vi "CalculateErrorOutLeftPosition__slk_mt.vi"(3 "add error configure":T2, 7 "position in":T1, 8 "error in (no error)":errorcluster, 11 "\"error in\" width":u32) -> (0 "error out":errorcluster, 5 "position out":T1)   [LabVIEW 2010, in "Lazyboots Menu Tool.lvlib"]
doc: "Gets error out left position."
uses:
  Library/Lazyboots Menu Tool.lvlib
  TypeDef/TypeDef_AddErrorConfigure__slk_mt.ctl
  <vilib>/Utility/miscctls.llb/LVPositionTypeDef.ctl
panel:
  # "CalculateErrorOutLeftPosition__slk_mt.vi\nGets error out left position.\n\nNOTICE -- YOU MUST LEAVE THIS NOTICE IN PLACE.\n\nCopyright (c) 2011, LIANG LIU Shawn.Liu.cn@gmail.com\nAll rights reserved.\n\nRedistribution and use in source and binary forms, with or without modification, are permitted provided that the following conditions are met:\n-Redistributions of source code must retain the above copyright notice, this list of conditions and the following disclaimer.\n-Redistributions in binary form must reproduce the above copyright notice, this list of conditions and the following disclaimer in the documentation and/or other materials provided with the distribution.\n-Neither the name of the eLp nor the names of its contributors may be used to endorse or promote products derived from this software without specific prior written permission.\n\nTHIS SOFTWARE IS PROVIDED BY THE COPYRIGHT HOLDERS AND CONTRIBUTORS \"AS IS\" AND ANY EXPRESS OR IMPLIED WARRANTIES, INCLUDING, BUT NOT LIMITED TO, THE IMPLIED WARRANTIES OF MERCHANTABILITY AND FITNESS FOR A PARTICULAR PURPOSE ARE DISCLAIMED. IN NO EVENT SHALL THE COPYRIGHT HOLDER OR CONTRIBUTORS BE LIABLE FOR ANY DIRECT, INDIRECT, INCIDENTAL, SPECIAL, EXEMPLARY, OR CONSEQUENTIAL DAMAGES (INCLUDING, BUT NOT LIMITED TO, PROCUREMENT OF SUBSTITUTE GOODS OR SERVICES; LOSS OF USE, DATA, OR PROFITS; OR BUSINESS INTERRUPTION) HOWEVER CAUSED AND ON ANY THEORY OF LIABILITY, WHETHER IN CONTRACT, STRICT LIABILITY, OR TORT (INCLUDING NEGLIGENCE OR OTHERWISE) ARISING IN ANY WAY OUT OF THE USE OF THIS SOFTWARE, EVEN IF ADVISED OF THE POSSIBILITY OF SUCH DAMAGE."
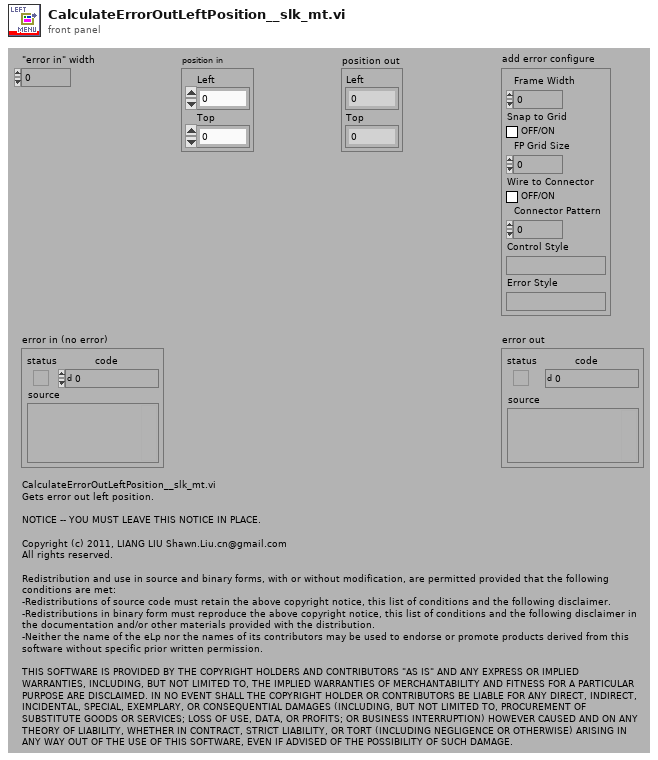
[diagram p1: front panel]
types:
  T1 = typedef "LVPositionTypeDef.ctl" = cluster{"Left":i32, "Top":i32}
  T2 = typedef "Lazyboots Menu Tool.lvlib/TypeDef_AddErrorConfigure__slk_mt.ctl" = cluster{"Frame Width":u32, "Snap to Grid":bool, "FP Grid Size":u32, "Wire to Connector":bool, "Connector Pattern":u32, "Control Style":string, "Error Style":string}
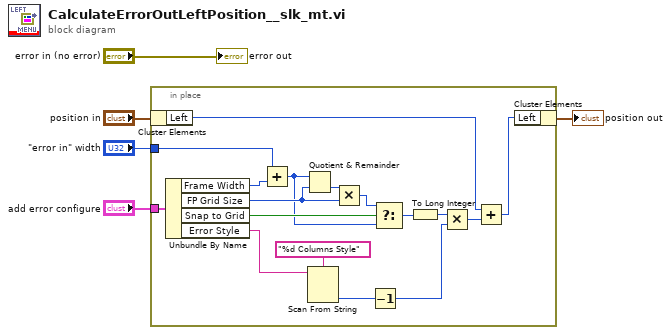
[diagram p0: block diagram]
diagram:
  n1 = in-place {
    in-place-border: "add error configure" -> [w22]
    in-place-border: "\"error in\" width" -> [w13]
    n2 = in-place-cluster #1("position in") -> ("Left"=w16:i32)
    n3 = Unbundle By Name(w22) -> ("Frame Width"=w15:u32, "FP Grid Size"=w14:u32, "Snap to Grid"=w8:bool, "Error Style"=w9:string)
    n4 = Add(x=w13, y=w15) -> (x+y=w7:u32)
    n5 = Quotient & Remainder(x=w7, y=w14) -> (floor(x/y)=w17:u32)  [unwired: 1 out]
    n6 = Scan From String(format string="%d Columns Style", input string=w9) -> (output 1=w19:i32)  [unwired: 3 in, 3 out]
    n7 = Multiply(x=w17, y=w14) -> (x*y=w10:u32)
    n8 = Decrement(x=w19) -> (x-1=w20:i32)
    n9 = Select(t=w10, s=w8, f=w7) -> (s? t:f=w11:u32)
    n10 = To Long Integer(number=w11) -> (32bit integer=w6:i32)
    n11 = Multiply(x=w6, y=w20) -> (x*y=w21:i32)
    n12 = Add(x=w16, y=w21) -> (x+y=w12:i32)
    n13 = in-place-cluster #1("Left"=w12) -> (→"position out":T1)
  }
  "error out" <- "error in (no error)"
